vi "SendInput String to Keys.vi"(8 "error in (no error)":errorcluster, 9 "ms Down/Up Duration (10)":u32=10, 10 "ms Press Duration (50)":u32=50, 11 "String":string) -> (0 "error out":errorcluster, 2 "Unknown keys?":bool, 3 "Keys":T1[](array[typedef]))   [LabVIEW 2026]
doc: "Returns an array of Virtual Key Codes from the printable keyboard String. \n(US keyboard support only)\n\nSupported Characters: \nabcdefghijklmnopqrstuvwxyz\nABCDEFGHIJKLMNOPQRSTUVWXYZ\n0123456789`~!@#$%^&*()-_=+[{]}\\|;:'\",<.>/?\n<space>\n\nCreated by: Ryan Pacini"
uses:
  labview_sendinput-master/SendInput/SendInput.llb/SendInput Event.ctl
  labview_sendinput-master/SendInput/SendInput.llb/SendInput Virtual Key Code.ctl
  labview_sendinput-master/SendInput/SendInput.llb/SendInput Key.ctl
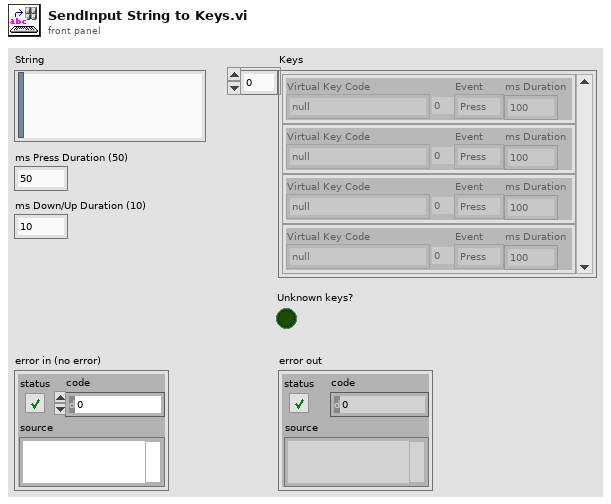
[diagram p1: front panel]
types:
  T1 = typedef "SendInput Key.ctl" = cluster{"Virtual Key Code":T2, "Event":T3, "ms Duration":u32}
  T2 = typedef "SendInput Virtual Key Code.ctl" = enum8{"null", "VK_LBUTTON", "VK_RBUTTON", "VK_CANCEL", "VK_MBUTTON", "VK_XBUTTON1", "VK_XBUTTON2", "0x07_Undefined", "VK_BACK", "VK_TAB", "0x0A_Reserved", "0x0B_Reserved", "VK_CLEAR", "VK_RETURN", "0x0E_Undefined", "0x0F_Undefined", "VK_SHIFT", "VK_CONTROL", "VK_MENU", "VK_PAUSE", "VK_CAPITAL", "VK_HANGUL", "0x16_Undefined", "VK_JUNJA", "VK_FINAL", "VK_HANJA", "0x1A_Undefined", "VK_ESCAPE", "VK_CONVERT", "VK_NONCONVERT", "VK_ACCEPT", "VK_MODECHANGE", "VK_SPACE", "VK_PRIOR", "VK_NEXT", "VK_END", "VK_HOME", "VK_LEFT", "VK_UP", "VK_RIGHT", "VK_DOWN", "VK_SELECT", "VK_PRINT", "VK_EXECUTE", "VK_SNAPSHOT", "VK_INSERT", "VK_DELETE", "VK_HELP", "0", "1", "2", "3", "4", "5", "6", "7", "8", "9", "0x3A_Undefined", "0x3B_Undefined", "0x3C_Undefined", "0x3D_Undefined", "0x3E_Undefined", "0x3F_Undefined", "0x40_Undefined", "A", "B", "C", "D", "E", "F", "G", "H", "I", "J", "K", "L", "M", "N", "O", "P", "Q", "R", "S", "T", "U", "V", "W", "X", "Y", "Z", "VK_LWIN", "VK_RWIN", "VK_APPS", "0x5E_Reserved", "VK_SLEEP", "VK_NUMPAD0", "VK_NUMPAD1", "VK_NUMPAD2", "VK_NUMPAD3", "VK_NUMPAD4", "VK_NUMPAD5", "VK_NUMPAD6", "VK_NUMPAD7", "VK_NUMPAD8", "VK_NUMPAD9", "VK_MULTIPLY", "VK_ADD", "VK_SEPARATOR", "VK_SUBTRACT", "VK_DECIMAL", "VK_DIVIDE", "VK_F1", "VK_F2", "VK_F3", "VK_F4", "VK_F5", "VK_F6", "VK_F7", "VK_F8", "VK_F9", "VK_F10", "VK_F11", "VK_F12", "VK_F13", "VK_F14", "VK_F15", "VK_F16", "VK_F17", "VK_F18", "VK_F19", "VK_F20", "VK_F21", "VK_F22", "VK_F23", "VK_F24", "0x88_Unassigned", "0x89_Unassigned", "0x8A_Unassigned", "0x8B_Unassigned", "0x8C_Unassigned", "0x8D_Unassigned", "0x8E_Unassigned", "0x8F_Unassigned", "VK_NUMLOCK", "VK_SCROLL", "0x92_OEM_Specific", "0x93_OEM_Specific", "0x94_OEM_Specific", "0x95_OEM_Specific", "0x96_OEM_Specific", "0x97_Unassigned", "0x98_Unassigned", "0x99_Unassigned", "0x9A_Unassigned", "0x9B_Unassigned", "0x9C_Unassigned", "0x9D_Unassigned", "0x9E_Unassigned", "0x9F_Unassigned", "VK_LSHIFT", "VK_RSHIFT", "VK_LCONTROL", "VK_RCONTROL", "VK_LMENU", "VK_RMENU", "VK_BROWSER_BACK", "VK_BROWSER_FORWARD", "VK_BROWSER_REFRESH", "VK_BROWSER_STOP", "VK_BROWSER_SEARCH", "VK_BROWSER_FAVORITES", "VK_BROWSER_HOME", "VK_VOLUME_MUTE", "VK_VOLUME_DOWN", "VK_VOLUME_UP", "VK_MEDIA_NEXT_TRACK", "VK_MEDIA_PREV_TRACK", "VK_MEDIA_STOP", "VK_MEDIA_PLAY_PAUSE", "VK_LAUNCH_MAIL", "VK_LAUNCH_MEDIA_SELECT", "VK_LAUNCH_APP1", "VK_LAUNCH_APP2", "0xB8_Reserved", "0xB9_Reserved", "VK_OEM_1", "VK_OEM_PLUS", "VK_OEM_COMMA", "VK_OEM_MINUS", "VK_OEM_PERIOD", "VK_OEM_2", "VK_OEM_3", "0xC1_Reserved", "0xC2_Reserved", "0xC3_Reserved", "0xC4_Reserved", "0xC5_Reserved", "0xC6_Reserved", "0xC7_Reserved", "0xC8_Reserved", "0xC9_Reserved", "0xCA_Reserved", "0xCB_Reserved", "0xCC_Reserved", "0xCD_Reserved", "0xCE_Reserved", "0xCF_Reserved", "0xD0_Reserved", "0xD1_Reserved", "0xD2_Reserved", "0xD3_Reserved", "0xD4_Reserved", "0xD5_Reserved", "0xD6_Reserved", "0xD7_Reserved", "0xD8_Reserved", "0xD9_Reserved", "0xDA_Reserved", "VK_OEM_4", "VK_OEM_5", "VK_OEM_6", "VK_OEM_7", "VK_OEM_8", "0xE0_Reserved", "0xE1_OEM_Specific", "VK_OEM_102", "0xE3_OEM_Specific", "0xE4_OEM_Specific", "VK_PROCESSKEY", "0xE6_OEM_Specific", "VK_PACKET", "0xE8_OEM_Specific", "0xE9_OEM_Specific", "0xEA_OEM_Specific", "0xEB_OEM_Specific", "0xEC_OEM_Specific", "0xED_OEM_Specific", "0xEE_OEM_Specific", "0xEF_OEM_Specific", "0xF0_OEM_Specific", "0xF1_OEM_Specific", "0xF2_OEM_Specific", "0xF3_OEM_Specific", "0xF4_OEM_Specific", "0xF5_OEM_Specific", "VK_ATTN", "VK_CRSEL", "VK_EXSEL", "VK_EREOF", "VK_PLAY", "VK_ZOOM", "VK_NONAME", "VK_PA1", "VK_OEM_CLEAR", "0xFF_Reserved"}
  T3 = typedef "SendInput Event.ctl" = enum8{"Press", "Down", "Up", "Wait"}
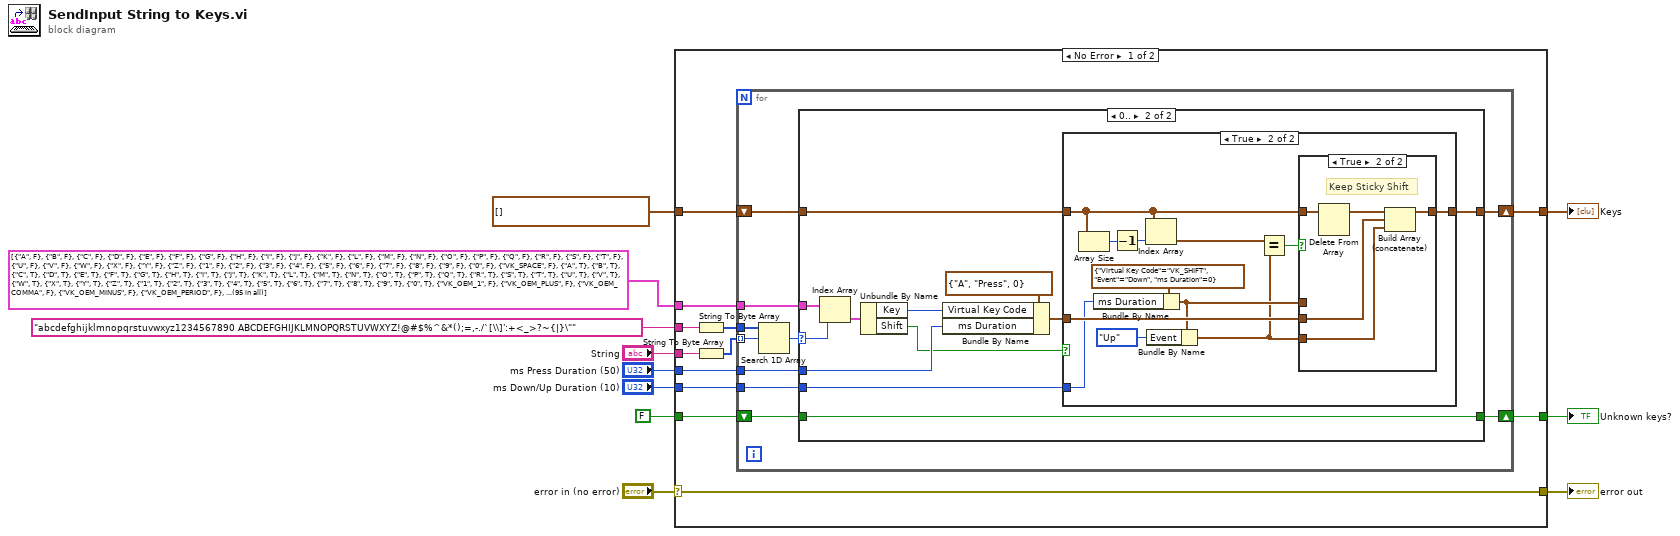
[diagram p0: block diagram]
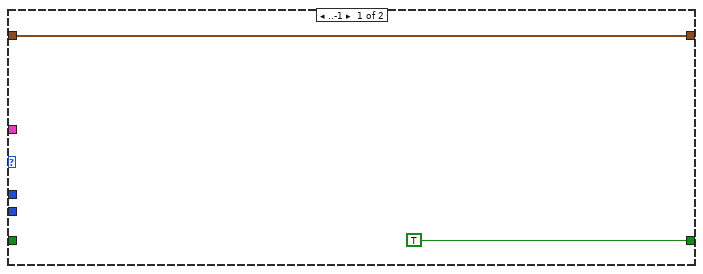
[diagram p2: hidden frame]
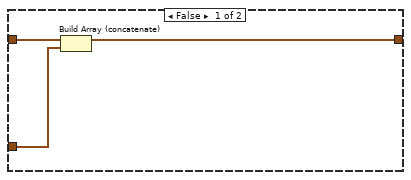
[diagram p3: hidden frame]
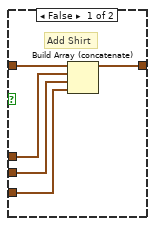
[diagram p4: hidden frame]
diagram:
  n1 = case shown="No Error" "error in (no error)" {
    selector: "error in (no error)" -> [w13 w75]
    tunnel: "String" -> [w23 _]
    tunnel: "abcdefghijklmnopqrstuvwxyz1234567890 ABCDEFGHIJKLMNOPQRSTUVWXYZ!@#$%^&*();=,-./`[\\]':+<_>?~{|}\"" ("concatenated string") -> [w22 _]
    tunnel: cluster{"Key":T2, "Shift":bool}[] [{"Key"=enum."A", "Shift"=FALSE}, {"Key"=enum."B", "Shift"=FALSE}, {"Key"=enum."C", "Shift"=FALSE}, {"Key"=enum."D", "Shift"=FALSE}, {"Key"=enum."E", "Shift"=FALSE}, {"Key"=enum."F", "Shift"=FALSE}, {"Key"=enum."G", "Shift"=FALSE}, {"Key"=enum."H", "Shift"=FALSE}, {"Key"=enum."I", "Shift"=FALSE}, {"Key"=enum."J", "Shift"=FALSE}, {"Key"=enum."K", "Shift"=FALSE}, {"Key"=enum."L", "Shift"=FALSE}, {"Key"=enum."M", "Shift"=FALSE}, {"Key"=enum."N", "Shift"=FALSE}, {"Key"=enum."O", "Shift"=FALSE}, {"Key"=enum."P", "Shift"=FALSE}, {"Key"=enum."Q", "Shift"=FALSE}, {"Key"=enum."R", "Shift"=FALSE}, {"Key"=enum."S", "Shift"=FALSE}, {"Key"=enum."T", "Shift"=FALSE}, {"Key"=enum."U", "Shift"=FALSE}, {"Key"=enum."V", "Shift"=FALSE}, {"Key"=enum."W", "Shift"=FALSE}, {"Key"=enum."X", "Shift"=FALSE}, {"Key"=enum."Y", "Shift"=FALSE}, {"Key"=enum."Z", "Shift"=FALSE}, {"Key"=enum."1", "Shift"=FALSE}, {"Key"=enum."2", "Shift"=FALSE}, {"Key"=enum."3", "Shift"=FALSE}, {"Key"=enum."4", "Shift"=FALSE}, {"Key"=enum."5", "Shift"=FALSE}, {"Key"=enum."6", "Shift"=FALSE}, {"Key"=enum."7", "Shift"=FALSE}, {"Key"=enum."8", "Shift"=FALSE}, {"Key"=enum."9", "Shift"=FALSE}, {"Key"=enum."0", "Shift"=FALSE}, {"Key"=enum."VK_SPACE", "Shift"=FALSE}, {"Key"=enum."A", "Shift"=TRUE}, {"Key"=enum."B", "Shift"=TRUE}, {"Key"=enum."C", "Shift"=TRUE}, {"Key"=enum."D", "Shift"=TRUE}, {"Key"=enum."E", "Shift"=TRUE}, {"Key"=enum."F", "Shift"=TRUE}, {"Key"=enum."G", "Shift"=TRUE}, {"Key"=enum."H", "Shift"=TRUE}, {"Key"=enum."I", "Shift"=TRUE}, {"Key"=enum."J", "Shift"=TRUE}, {"Key"=enum."K", "Shift"=TRUE}, {"Key"=enum."L", "Shift"=TRUE}, {"Key"=enum."M", "Shift"=TRUE}, {"Key"=enum."N", "Shift"=TRUE}, {"Key"=enum."O", "Shift"=TRUE}, {"Key"=enum."P", "Shift"=TRUE}, {"Key"=enum."Q", "Shift"=TRUE}, {"Key"=enum."R", "Shift"=TRUE}, {"Key"=enum."S", "Shift"=TRUE}, {"Key"=enum."T", "Shift"=TRUE}, {"Key"=enum."U", "Shift"=TRUE}, {"Key"=enum."V", "Shift"=TRUE}, {"Key"=enum."W", "Shift"=TRUE}, {"Key"=enum."X", "Shift"=TRUE}, {"Key"=enum."Y", "Shift"=TRUE}, {"Key"=enum."Z", "Shift"=TRUE}, {"Key"=enum."1", "Shift"=TRUE}, {"Key"=enum."2", "Shift"=TRUE}, {"Key"=enum."3", "Shift"=TRUE}, {"Key"=enum."4", "Shift"=TRUE}, {"Key"=enum."5", "Shift"=TRUE}, {"Key"=enum."6", "Shift"=TRUE}, {"Key"=enum."7", "Shift"=TRUE}, {"Key"=enum."8", "Shift"=TRUE}, {"Key"=enum."9", "Shift"=TRUE}, {"Key"=enum."0", "Shift"=TRUE}, {"Key"=enum."VK_OEM_1", "Shift"=FALSE}, {"Key"=enum."VK_OEM_PLUS", "Shift"=FALSE}, {"Key"=enum."VK_OEM_COMMA", "Shift"=FALSE}, {"Key"=enum."VK_OEM_MINUS", "Shift"=FALSE}, {"Key"=enum."VK_OEM_PERIOD", "Shift"=FALSE}, {"Key"=enum."VK_OEM_2", "Shift"=FALSE}, {"Key"=enum."VK_OEM_3", "Shift"=FALSE}, {"Key"=enum."VK_OEM_4", "Shift"=FALSE}, {"Key"=enum."VK_OEM_5", "Shift"=FALSE}, {"Key"=enum."VK_OEM_6", "Shift"=FALSE}, {"Key"=enum."VK_OEM_7", "Shift"=FALSE}, {"Key"=enum."VK_OEM_1", "Shift"=TRUE}, {"Key"=enum."VK_OEM_PLUS", "Shift"=TRUE}, {"Key"=enum."VK_OEM_COMMA", "Shift"=TRUE}, {"Key"=enum."VK_OEM_MINUS", "Shift"=TRUE}, {"Key"=enum."VK_OEM_PERIOD", "Shift"=TRUE}, {"Key"=enum."VK_OEM_2", "Shift"=TRUE}, {"Key"=enum."VK_OEM_3", "Shift"=TRUE}, {"Key"=enum."VK_OEM_4", "Shift"=TRUE}, {"Key"=enum."VK_OEM_5", "Shift"=TRUE}, {"Key"=enum."VK_OEM_6", "Shift"=TRUE}, {"Key"=enum."VK_OEM_7", "Shift"=TRUE}] ("appended array 4") -> [w19 _]
    tunnel: "ms Press Duration (50)" -> [w18 _]
    tunnel: "ms Down/Up Duration (10)" -> [w17 _]
    tunnel: [w16 w74] -> w8
    tunnel: [w15 w73] -> w7
    tunnel: T1[] [] -> [w14 w74]
    tunnel: [w13 w75] -> w5
    tunnel: FALSE -> [w12 w73]
    frame No Error {
      n2 = String To Byte Array(string=w22) -> (unsigned byte array=w21:u8[])
      n3 = String To Byte Array(string=w23) -> (unsigned byte array=w20:u8[])
      n4 = for {
        tunnel: w21 -> [w33]
        tunnel: w20 -> [w32] mode=indexing
        tunnel: w19 -> [w30]
        tunnel: w18 -> [w29]
        tunnel: w17 -> [w28]
        shift-right: [w25] -> w15
        shift-left: w12 -> [w26]
        shift-right: [w27] -> w16
        shift-left: w14 -> [w24]
        n5 = Search 1D Array(1D array=w33, element=w32) -> (index of element=w31:i32)  [unwired: 1 in]
        n6 = case shown="0.." w31 {
          selector: w31 -> [_ w47]
          tunnel: w30 -> [_ w46]
          tunnel: w29 -> [_ w42]
          tunnel: w28 -> [_ w40]
          tunnel: [w34 w38] -> w27
          tunnel: w26 -> [_ w37]
          tunnel: [TRUE w37] -> w25
          tunnel: w24 -> [w34 w36]
          frame ..-1 {
          }
          frame 0.. {
            n7 = Index Array(array=w46, index=w47) -> (element=w45:cluster{"Key":T2, "Shift":bool})
            n8 = Unbundle By Name(w45) -> ("Key"=w43:T2, "Shift"=w39:bool)
            n9 = Bundle By Name(cluster=T1 {"Virtual Key Code"=enum."A", "Event"=enum."Press", "ms Duration"=0} ("Key"), "Virtual Key Code"=w43, "ms Duration"=w42) -> (w41:T1)
            n10 = case shown="True" w39 {
              tunnel: w41 -> [w50 w62]
              tunnel: w40 -> [_ w60]
              tunnel: [w49 w57] -> w38
              tunnel: w36 -> [w48 w52]
              frame False {
                n11 = Build Array (concatenate)(w48, w50) -> (w49:T1[])
              }
              frame True {
                n12 = Array Size(array=w52) -> (size(s)=w56:i32)
                n13 = Bundle By Name(cluster=T1 {"Virtual Key Code"=enum."VK_SHIFT", "Event"=enum."Down", "ms Duration"=0} ("Key"), "ms Duration"=w60) -> (w58:T1)
                n14 = Decrement(x=w56) -> (x-1=w55:i32)
                n15 = Index Array(array=w52, index=w55) -> (element=w54:T1)
                n16 = Bundle By Name(cluster=w58, "Event"=SendInput_Event."Up") -> (w53:T1)
                n17 = Equal?(x=w54, y=w53) -> (x = y?=w51:bool)
                n18 = case shown="True" w51 {
                  tunnel: w62 -> [w67 w69]
                  tunnel: w58 -> [w66 _]
                  tunnel: [w65 w70] -> w57
                  tunnel: w53 -> [w64 w68]
                  tunnel: w52 -> [w63 w72]
                  frame False {
                    # "Add Shirt"
                    n19 = Build Array (concatenate)(w63, w66, w67, w64) -> (w65:T1[])
                  }
                  frame True {
                    # "Keep Sticky Shift"
                    n20 = Delete From Array(array=w72) -> (array with subset deleted=w71:T1[])  [unwired: 2 in, 1 out]
                    n21 = Build Array (concatenate)(w71, w69, w68) -> (w70:T1[])
                  }
                }
              }
            }
          }
        }
      }
    }
    frame Error {
    }
  }
  "Keys" <- w8
  "Unknown keys?" <- w7
  "error out" <- w5
